vi "Create Graph from Solution(Schedule).vi"(6 "Job Order for Machines":u16[][](array[numeric])=[[0, 6, 3], [7, 4, 1], [5, 8, 2]], 7 "Machine Order for Jobs":u16[][](array[numeric])=[[0, 2, 1], [5, 4, 3], [7, 8, 6]], 8 "error in (no error)":errorcluster, 9 "Number of Machines":u8, 10 "Number of Jobs":u8, 11 "Graph.lvclass":refnum<class "Graph.lvclass">) -> (0 "error out":errorcluster, 3 "Graph out":refnum<class "Graph.lvclass">)   [LabVIEW 2013, in "Graph.lvclass"]
uses:
  Graph.lvclass
  Graph.lvclass/Graph.ctl
panel:
  out "Starting Vertices":i32[](array[numeric])
  out "Unique Values of Dictionary":u16[](array[numeric])
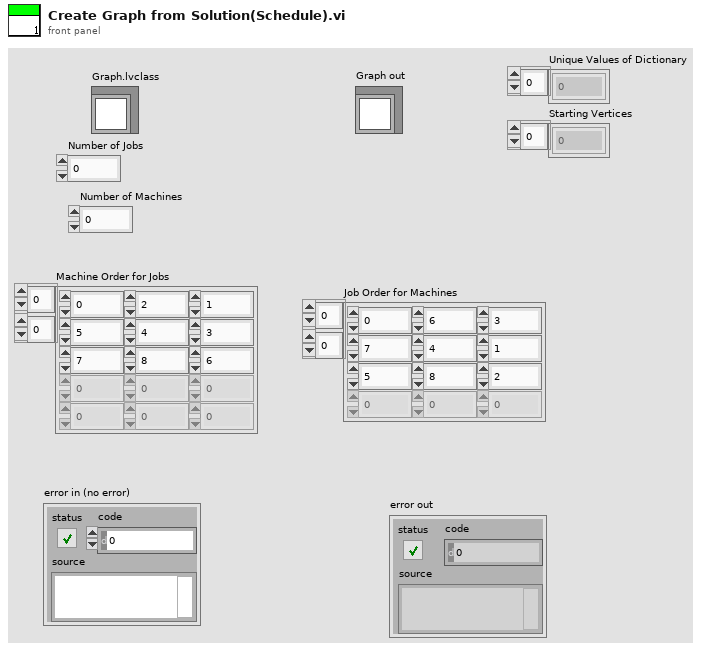
[diagram p1: front panel]
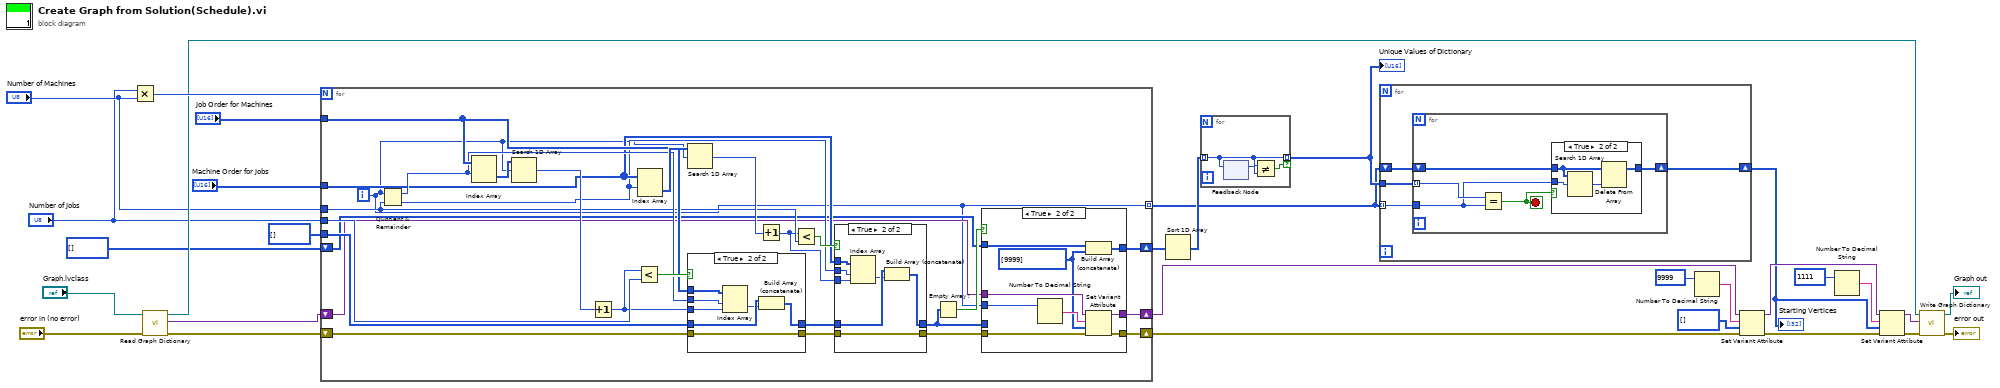
[diagram p0: block diagram]
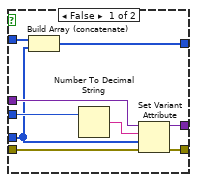
[diagram p3: hidden frame]
diagram:
  n1 = Multiply(x="Number of Jobs", y="Number of Machines") -> (x*y=w30:u8)
  n2 = call "Read Graph Dictionary.vi"("error in (no error)"="error in (no error)", "Graph in"="Graph.lvclass") -> ("error out"=w25:errorcluster, "Graph Dictionary"=w26:variant, "Graph out"=w22:refnum<class "Graph.lvclass">)  [unwired: 7 in]
  n3 = for {
    N: w30 -> [_]
    tunnel: "Job Order for Machines" -> [w49]
    tunnel: "Machine Order for Jobs" -> [w42]
    tunnel: "Number of Machines" -> [w44]
    shift-right: [w35] -> w20
    shift-left: w26 -> [w36]
    shift-right: [w38] -> w19
    shift-left: w25 -> [w55]
    tunnel: u16[] [] -> [w53]
    tunnel: "Number of Jobs" -> [w51]
    shift-right: [w32] -> w14
    shift-left: u16[] [] -> [w33]
    tunnel: [w31] -> w12 mode=indexing
    i -> [w31]
    n4 = Quotient & Remainder(x=w31, y=w44) -> (x-y*floor(x/y)=w48:i32, floor(x/y)=w41:i32)
    n5 = Index Array(array=w49, index (row)=w48) -> (element=w57:u16[])  [unwired: 1 in]
    n6 = Search 1D Array(1D array=w57, element=w31) -> (index of element=w52:i32)  [unwired: 1 in]
    n7 = Increment(x=w52) -> (x+1=w47:i32)
    n8 = Less?(x=w47, y=w51) -> (x < y?=w50:bool)
    n9 = Index Array(array=w42, index (row)=w41) -> (element=w56:u16[])  [unwired: 1 in]
    n10 = Search 1D Array(1D array=w56, element=w31) -> (index of element=w45:i32)  [unwired: 1 in]
    n11 = case shown="True" w50 {
      tunnel: w55 -> [w86 w93]
      tunnel: [w86 w93] -> w54
      tunnel: w53 -> [w85 w89]
      tunnel: w49 -> [_ w92]
      tunnel: w48 -> [_ w91]
      tunnel: w47 -> [_ w90]
      tunnel: [w85 w87] -> w46
      frame False {
      }
      frame True {
        n12 = Index Array(array=w92, index (row)=w91, index (col)=w90) -> (element=w88:u16)
        n13 = Build Array (concatenate)(w89, w88) -> (w87:u16[])
      }
    }
    n14 = Increment(x=w45) -> (x+1=w40:i32)
    n15 = Less?(x=w40, y=w44) -> (x < y?=w43:bool)
    n16 = case shown="True" w43 {
      tunnel: w54 -> [w77 w84]
      tunnel: [w77 w84] -> w39
      tunnel: w46 -> [w76 w80]
      tunnel: w42 -> [_ w81]
      tunnel: w41 -> [_ w83]
      tunnel: w40 -> [_ w82]
      tunnel: [w76 w78] -> w34
      frame False {
      }
      frame True {
        n17 = Index Array(array=w81, index (row)=w83, index (col)=w82) -> (element=w79:u16)
        n18 = Build Array (concatenate)(w80, w79) -> (w78:u16[])
      }
    }
    n19 = Empty Array?(array=w34) -> (empty?=w37:bool)
    n20 = case shown="True" w37 {
      tunnel: w39 -> [w65 w72]
      tunnel: [w64 w71] -> w38
      tunnel: w36 -> [w66 w75]
      tunnel: w31 -> [w62 w74]
      tunnel: [w63 w70] -> w35
      tunnel: w34 -> [w59 _]
      tunnel: w33 -> [w60 w69]
      tunnel: [w58 w68] -> w32
      frame False {
        n21 = Build Array (concatenate)(w60, w59) -> (w58:u16[])
        n22 = Number To Decimal String(number=w62) -> (decimal integer string=w61:string)  [unwired: 1 in]
        n23 = Set Variant Attribute(Variant=w66, name=w61, value=w59, error in=w65) -> (Variant out=w63:variant, error out=w64:errorcluster)  [unwired: 1 out]
      }
      frame True {
        w67 = u16[] [9999]
        n24 = Number To Decimal String(number=w74) -> (decimal integer string=w73:string)  [unwired: 1 in]
        n25 = Build Array (concatenate)(w69, w67) -> (w68:u16[])
        n26 = Set Variant Attribute(Variant=w75, name=w73, value=w67, error in=w72) -> (Variant out=w70:variant, error out=w71:errorcluster)  [unwired: 1 out]
      }
    }
  }
  n27 = Sort 1D Array(array=w14) -> (sorted array=w15:u16[])
  n28 = for {
    tunnel: w15 -> [w95] mode=indexing
    tunnel: [w95] -> w13 mode=indexing if=w94
    n29 = feedback-in #1(w95) -> ()
    n30 = feedback #1() -> (w96:u16)  [unwired: 1 in]
    n31 = Not Equal?(x=w95, y=w96) -> (x != y?=w94:bool)
  }
  "Unique Values of Dictionary" <- w13
  n32 = for {
    tunnel: w13 -> [w100]
    tunnel: w12 -> [w99] mode=indexing
    shift-right: [w97] -> w4
    shift-left: w12 -> [w98]
    n33 = for {
      tunnel: w100 -> [w105] mode=indexing
      tunnel: w99 -> [w101]
      shift-right: [w103] -> w97
      shift-left: w98 -> [w104]
      stop <- w102 stop-if-true
      n34 = Equal?(x=w105, y=w101) -> (x = y?=w102:bool)
      n35 = case shown="True" w102 {
        tunnel: w104 -> [w106 w109]
        tunnel: [w106 w110] -> w103
        tunnel: w101 -> [_ w108]
        frame False {
        }
        frame True {
          n36 = Search 1D Array(1D array=w109, element=w108) -> (index of element=w107:i32)  [unwired: 1 in]
          n37 = Delete From Array(array=w109, index=w107) -> (array with subset deleted=w110:i32[])  [unwired: 1 in, 1 out]
        }
      }
    }
  }
  "Starting Vertices" <- w4
  n38 = Number To Decimal String(number=u16 9999) -> (decimal integer string=w17:string)  [unwired: 1 in]
  n39 = Set Variant Attribute(Variant=w20, name=w17, value=u16[] [], error in=w19) -> (Variant out=w8:variant, error out=w7:errorcluster)  [unwired: 1 out]
  n40 = Number To Decimal String(number=1111) -> (decimal integer string=w5:string)  [unwired: 1 in]
  n41 = Set Variant Attribute(Variant=w8, name=w5, value=w4, error in=w7) -> (Variant out=w2:variant, error out=w3:errorcluster)  [unwired: 1 out]
  n42 = call "Write Graph Dictionary.vi"("error in (no error)"=w3, "Graph Dictionary"=w2, "Graph in"=w22) -> ("error out"=→"error out":errorcluster, "Graph out"=→"Graph out":refnum<class "Graph.lvclass">)  [unwired: 7 in]
